vi "PH_PILS.PC _Enabling Laser changed.vi"(0 "i ref in":refnum<vi>, 5 "error in":errorcluster) -> (14 "i ref out":refnum<vi>, 19 "error out":errorcluster)   [LabVIEW 2014, in "PH_PILS.lvlib"]
uses:
  PH_PILS.lvlib
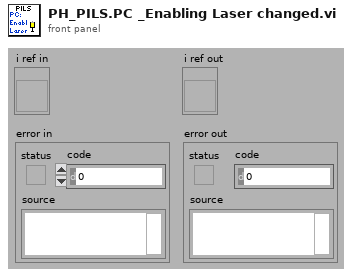
[diagram p1: front panel]
types:
  T1 = enum16{"unknown", "intern", "4 (Z6)", "3", "2", "1"}[]
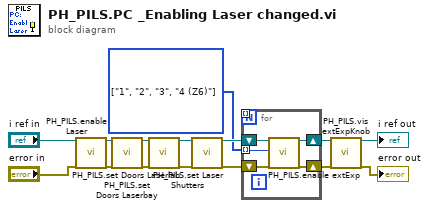
[diagram p0: block diagram]
diagram:
  w1 = T1 [enum."1", enum."2", enum."3", enum."4 (Z6)"] items=["unknown", "intern", "4 (Z6)", "3", "2", "1"]
  n1 = call "PH_PILS.enable Laser.vi"("i ref in"="i ref in", "error in"="error in") -> ("i ref out"=w13:refnum<vi>, "error out"=w11:errorcluster)  [unwired: 16 in]
  n2 = call "PH_PILS.set Doors Laserbay.vi"("i ref in"=w13, "error in"=w11) -> ("i ref out"=w12:refnum<vi>, "error out"=w10:errorcluster)  [unwired: 16 in]
  n3 = call "PH_PILS.set Doors Laserlab.vi"("i ref in"=w12, "error in"=w10) -> ("i ref out"=w14:refnum<vi>, "error out"=w15:errorcluster)  [unwired: 16 in]
  n4 = call "PH_PILS.set Laser Shutters.vi"("i ref in"=w14, "error in"=w15) -> ("i ref out"=w3:refnum<vi>, "error out"=w5:errorcluster)  [unwired: 16 in]
  n5 = for {
    N -> [w16]
    shift-right: [w18] -> w2
    shift-left: w3 -> [w19]
    shift-right: [w20] -> w4
    shift-left: w5 -> [w21]
    tunnel: w1 -> [w17] mode=indexing
    tunnel: [w16] -> _ mode=indexing
    n6 = call "PH_PILS.enable extExp.vi"("i ref in"=w19, "Experiment.Experiment"=w17, "error in"=w21) -> ("i ref out"=w18:refnum<vi>, "error out"=w20:errorcluster)  [unwired: 15 in]
  }
  n7 = call "PH_PILS.vis extExpKnob.vi"("i ref in"=w2, "error IO"=w4) -> ("i ref out"=→"i ref out":refnum<vi>, "error out"=→"error out":errorcluster)  [unwired: 16 in]
